vi "SV Continuous Swept-Sine Frequency Response.vi"(0 "scaled signals [EU]":waveform(dbl)[](array[waveform]), 1 "view":T3={"dB on? (T)"=TRUE, "unwrap phase? (F)"=FALSE, "convert to degree? (T)"=TRUE}, 2 "reset? (F)":bool, 5 "reference channel":i32=-1, 11 "error in (no error)":errorcluster, 12 "buffer settings":T2 {"buffer mode" items=["Infinite length", "Last block data", "Custom"]}, 13 "zero delay? (F)":bool) -> (3 "unit labels":T1(array[cluster]), 4 "scaled signals out [EU]":waveform(dbl)[](array[waveform]), 6 "magnitudes":cluster{"frequency":dbl[], "magnitude":dbl[]}[](array[cluster]) {"magnitude" format="%.2f"; "frequency" format="%.2f"}, 8 "phases":cluster{"frequency":dbl[], "phase":dbl[]}[](array[cluster]) {"phase" format="%.2f"; "frequency" format="%.2f"}, 15 "error out":errorcluster)   [LabVIEW 2017, in "SoundVib_ContSweptSine.lvlib"]
doc: "Computes frequency response measurements, including magnitudes and phases, by performing a continuous swept-sine measurement."
uses:
  <vilib>/addons/Sound and Vibration/svt_Continuous Swept Sine/SoundVib_ContSweptSine.lvlib
  <vilib>/addons/_NISVFA/_Shared subVIs/Controls/sv_Buffer XY Settings.ctl
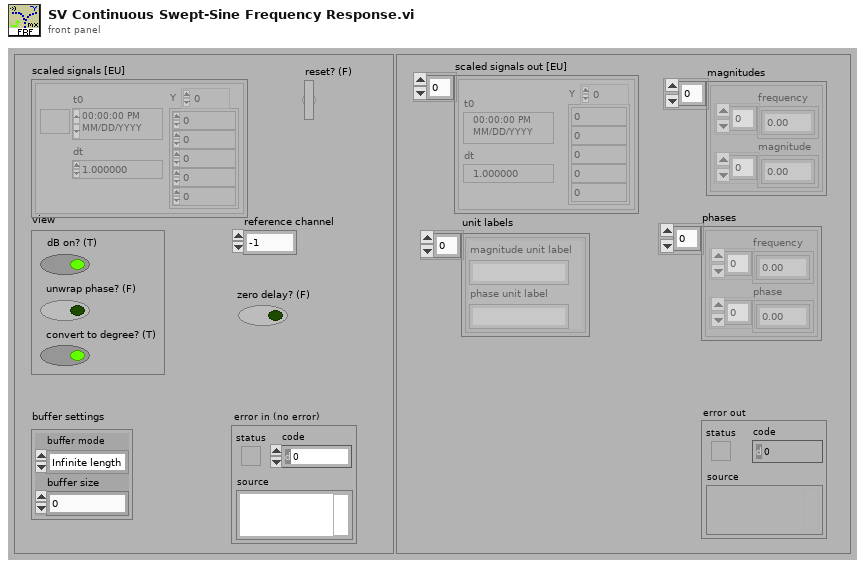
[diagram p1: front panel]
types:
  T1 = cluster{"magnitude unit label":string, "phase unit label":string}[]
  T2 = typedef "sv_Buffer XY Settings.ctl" = cluster{"buffer mode":u16, "buffer size":dbl}
  T3 = cluster{"dB on? (T)":bool, "unwrap phase? (F)":bool, "convert to degree? (T)":bool}
  T4 = typedef "svc_Resampled Channel Info.ctl" = cluster{"channel name":string, "description":string, " channel info":T5}
  T5 = typedef "svc_Channel Info.ctl" = cluster{"sensor sensitivity":dbl, "engineering units":T6, "dB reference":dbl, "custom label":string, "weighting filter":T7, "pregain":dbl}
  T6 = typedef "svc_Engineering Units Text Ring.ctl" = u16
  T7 = typedef "svc_Weighting Filter Text Ring.ctl" = u16
  T8 = typedef "OAT Position Info.ctl" = cluster{"positions [s]":dbl[], "samples/rev":dbl}
  T9 = cluster{"time/rev/freq":dbl[], "magnitude":dbl[]}[][]
  T10 = cluster{"time/rev/freq":dbl[], "phase":dbl[]}[][]
  T11 = cluster{"time/rev/freq":dbl[], "magnitude":dbl[]}[]
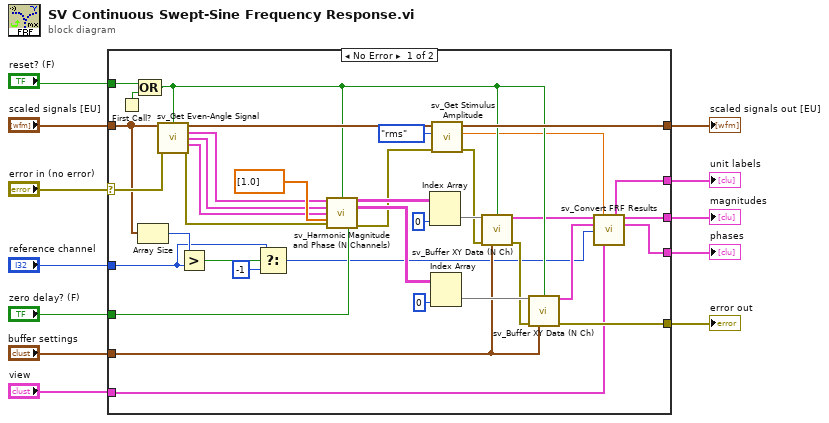
[diagram p0: block diagram]
diagram:
  n1 = case shown="No Error" "error in (no error)" {
    selector: "error in (no error)" -> [w44 w51]
    tunnel: [w26 w51] -> w11
    tunnel: "view" -> [w22 _]
    tunnel: [w19 _] -> w10
    tunnel: "scaled signals [EU]" -> [w18 w50]
    tunnel: [w33 w50] -> w9
    tunnel: [w21 _] -> w8
    tunnel: "reference channel" -> [w14 _]
    tunnel: "buffer settings" -> [w27 _]
    tunnel: "zero delay? (F)" -> [w36 _]
    tunnel: "reset? (F)" -> [w34 _]
    tunnel: [w20 _] -> w1
    frame No Error {
      n2 = First Call?() -> (First Call?: T/F=w35:bool)
      n3 = Array Size(array=w18) -> (size(s)=w17:i32)
      n4 = Compound Arithmetic op=OR(w34, w35) -> (w29:bool)
      n5 = call <vilib>:"sv_Get Even-Angle Signal.vi"("data to process"=w18, "reset?"=w29, "error in (no error)"=w44) -> ("data to process out"=w37:waveform(dbl)[], "even-angle signals"=w43:cluster{"r0":dbl, "dr":dbl, "Y":dbl[]}[], "even-angle channel info"=w42:T4[], "even-angle position info"=w41:T8, "error out"=w40:errorcluster)  [unwired: 7 in, 1 out]
      n6 = Greater?(x=w17, y=w14) -> (0:w16:bool)
      n7 = Select(t=w14, s=w16, f=-1) -> (s? t:f=w13:i32)
      n8 = call <vilib>:"sv_Harmonic Magnitude and Phase (N Channels).vi"("even-angle signals"=w43, "reset? (F)"=w29, "even-angle channel info"=w42, "even-angle position info"=w41, "orders to compute (1.0)"=dbl[] [1.0], "error in (no error)"=w40, "zero delay? (F)"=w36) -> ("magnitudes [RMS]"=w48:T9, "phases [phase lag]"=w45:T10, "error out"=w39:errorcluster)  [unwired: 5 in, 1 out]
      n9 = Index Array(array=w48, index (col)=0 ("disabled index (col)")) -> (element=w32:T11)  [unwired: 1 in]
      n10 = Index Array(array=w45, index (col)=0 ("disabled index (col)")) -> (element=w30:cluster{"time/rev/freq":dbl[], "phase":dbl[]}[])  [unwired: 1 in]
      n11 = call <vilib>:"sv_Get Stimulus Amplitude.vi"("error in (no error)"=w39, "view"=enum16{"rms", "peak", "peak-peak"}."rms", "data to process"=w37) -> ("error out"=w31:errorcluster, "amplitude [V]"=w24:dbl, "data to process out"=w33:waveform(dbl)[])  [unwired: 6 in]
      n12 = call <vilib>:"sv_Buffer XY Data (N Ch).vi"("XY signals"=w32, "reset? (F)"=w29, "error in (no error)"=w31, "buffer settings"=w27) -> ("buffered XY signals"=w25:cluster{"X":dbl[], "Y":dbl[]}[], "error out"=w28:errorcluster)  [unwired: 10 in]
      n13 = call <vilib>:"sv_Buffer XY Data (N Ch).vi"("XY signals"=w30, "reset? (F)"=w29, "error in (no error)"=w28, "buffer settings"=w27) -> ("buffered XY signals"=w23:cluster{"X":dbl[], "Y":dbl[]}[], "error out"=w26:errorcluster)  [unwired: 10 in]
      n14 = call <vilib>:"sv_Convert FRF Results.vi"("magnitudes"=w25, "ref amplitude"=w24, "Phases"=w23, "reference channel"=w13, "view"=w22) -> ("Units"=w20:cluster{string, string}[], "Magnitudes"=w21:cluster{"X":dbl[], "Y":dbl[]}[], "Phases"=w19:cluster{"X":dbl[], "Y":dbl[]}[])  [unwired: 8 in]
    }
    frame Error {
    }
  }
  "error out" <- w11
  "magnitudes" <- w8
  "phases" <- w10
  "scaled signals out [EU]" <- w9
  "unit labels" <- w1
